vi "akcelerometrWykres.vi"() -> ()   [LabVIEW 2014]
uses:
  <vilib>/MakerHub/LINX/Public/Utilities/Open Local.vi
  <vilib>/MakerHub/LINX/LMH-LINX.lvlib
panel:
  out "deleted portion":dbl[][](array[numeric])
  out "size(s)":i32
  out "Waveform Graph":dbl[][](graph)
  in  "stop":bool
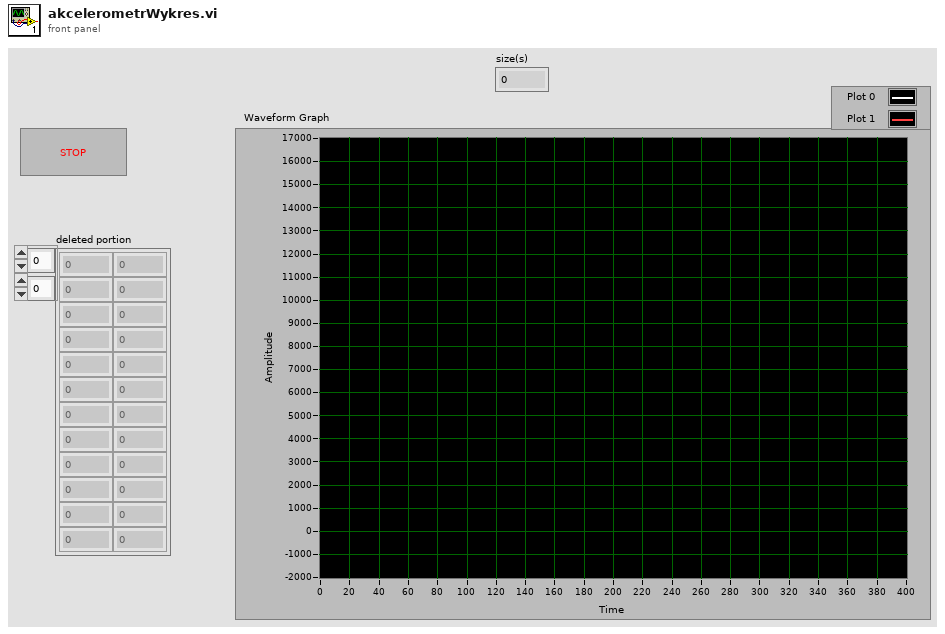
[diagram p1: front panel]
types:
  T1 = typedef "LMH-LINX.lvlib/LINX Ref.ctl" = cluster{"IO":T2, "Interface":T3, "LINX Device Config":T4}
  T2 = typedef "LMH-LINX.lvlib/Platform.ctl" = enum16{"Remote", "Local"}
  T3 = typedef "LMH-LINX.lvlib/Interface.ctl" = enum16{"Serial", "TCP"}
  T4 = typedef "LMH-LINX.lvlib/Device.lvlib/LINX Device Config.ctl" = cluster{"Interface":T3, "COM Port":refnum<visa-resource-name>, "TCP Configuration":T5, "Device Family":u8, "Device ID":u8, "Device Name":string, "TCP Ref":refnum<k5>, "Channels":T6}
  T5 = typedef "LMH-LINX.lvlib/Device.lvlib/TCP Config.ctl" = cluster{"IP Address":string, "Port":u16}
  T6 = typedef "LMH-LINX.lvlib/Channels.ctl" = cluster{"DI":u8[], "DO":u8[], "AI":u8[], "AO":u8[], "PWM":u8[], "QE":u8[], "UART":u8[], "I2C 2":u8[], "SPI":u8[], "CAN":u8[], "Servo":u8[], "AI Ref (V)":dbl, "AI Resolution (Bits)":u8, "AO Ref (V)":dbl, "AO Resolution (Bits)":u8}
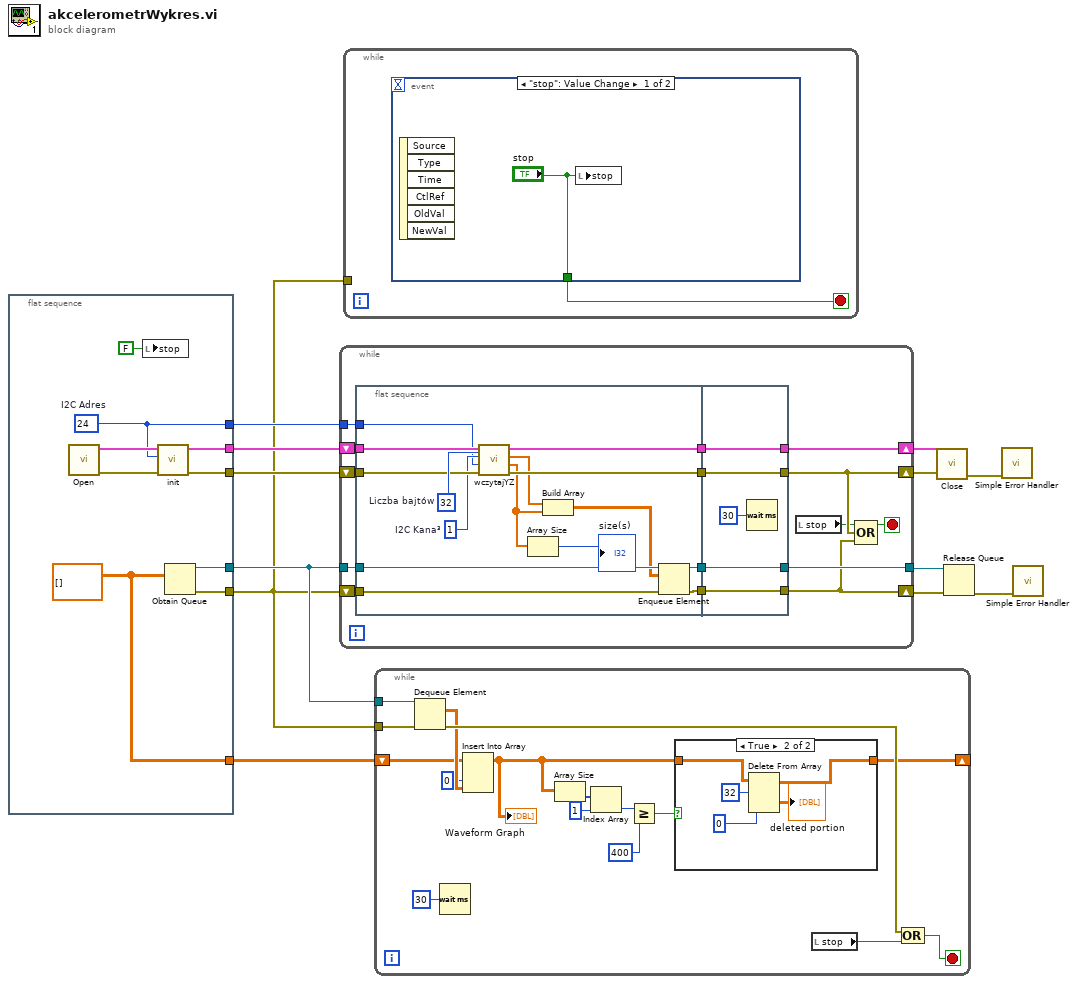
[diagram p0: block diagram]
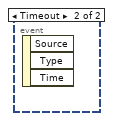
[diagram p2: hidden frame]
diagram:
  n1 = flat-sequence {
    tunnel: [w21] -> w12
    tunnel: [w20] -> w2
    tunnel: [w17] -> w9
    tunnel: [w16] -> w4
    tunnel: [w15] -> w1
    tunnel: [w13] -> w3
    frame #0 {
      w13 = dbl[][] [] ("appended array")
      w17 = u8 24  # I2C Adres
      n2 = call-poly <vilib>:"Open.vi"() -> ("Error Out"=w18:errorcluster, "LINX Resource"=w19:T1)  [unwired: 9 in, 1 out]
      n3 = local write "stop"(FALSE ("stop")) -> ()
      n4 = call "init.vi"("Error In"=w18, "I2C Adres"=w17, "LINX Ref"=w19) -> ("Error Out"=w20:errorcluster, "LINX Resource"=w21:T1)  [unwired: 7 in]
      n5 = Obtain Queue(element data type=w13) -> (queue out=w16:refnum<queue>, error out=w15:errorcluster)  [unwired: 4 in, 1 out]
    }
  }
  n6 = while {
    tunnel: w9 -> [w33]
    shift-right: [w34] -> w11
    shift-left: w12 -> [w36]
    shift-right: [w31] -> w10
    shift-left: w2 -> [w35]
    tunnel: w4 -> [w30]
    tunnel: [w28] -> w7
    shift-right: [w27] -> w6
    shift-left: w1 -> [w29]
    stop <- w32 stop-if-true
    n7 = flat-sequence {
      tunnel: w36 -> [w50]
      tunnel: w35 -> [w49]
      tunnel: w33 -> [w46]
      tunnel: w30 -> [w44]
      tunnel: w29 -> [w43]
      tunnel: [w47] -> w25
      tunnel: [w45] -> w24
      tunnel: [w42] -> w23
      tunnel: [w41] -> w22
      tunnel: [w53] -> w27
      tunnel: [w54] -> w28
      tunnel: [w55] -> w31
      tunnel: [w56] -> w34
      tunnel: w25 -> [w56]
      tunnel: w24 -> [w55]
      tunnel: w23 -> [w54]
      tunnel: w22 -> [w53]
      frame #0 {
        w48 = u8 1  # I2C Kana³
        w51 = u8 32  # Liczba bajtów
        n8 = call "wczytajYZ.vi"("Liczba bajtów"=w51, "error in (no error)"=w49, "I2C Adres"=w46, "I2C Kana³"=w48, "LINX Resource in"=w50) -> ("error out"=w45:errorcluster, "Oœ Z"=w38:dbl[], "Oœ Y"=w39:dbl[], "LINX Resource out"=w47:T1)  [unwired: 3 in]
        n9 = Array Size(array=w38) -> (size(s)=→"size(s)":i32)
        n10 = Build Array(w39, w38) -> (w40:dbl[][])
        n11 = Enqueue Element(queue=w44, element=w40, error in (no error)=w43) -> (queue out=w42:refnum<queue>, error out=w41:errorcluster)  [unwired: 1 in, 1 out]
      }
      frame #1 {
        n12 = Wait (ms)(milliseconds to wait=u32 30 ("millisecond multiple")) -> ()  [unwired: 1 out]
      }
    }
    n13 = local read "stop"() -> (w26:bool)
    n14 = Compound Arithmetic op=OR(w26, w31, w27) -> (w32:bool)
  }
  n15 = while {
    tunnel: w1 -> [_]
    stop <- w57 stop-if-true
    n16 = event shown="[0] \"stop\": Value Change" {
      selector: _ -> [_ _]
      dyn-events: _ -> [_ _]
      timeout: _ -> [_ _]
      tunnel: ["stop" _] -> w57
      event "stop": Value Change {
        n17 = event-data() -> ()  [unwired: 1 in, 6 out]
        n18 = local write "stop"("stop") -> ()
      }
      event Timeout {
        n19 = event-data() -> ()  [unwired: 1 in, 3 out]
      }
    }
  }
  n20 = while {
    tunnel: w4 -> [w74]
    tunnel: w1 -> [w73]
    shift-right: [w66] -> _
    shift-left: w3 -> [w68]
    stop <- w71 stop-if-true
    n21 = Dequeue Element(queue=w74, error in (no error)=w73) -> (element=w69:dbl[][], error out=w70:errorcluster)  [unwired: 1 in, 2 out]
    n22 = Wait (ms)(milliseconds to wait=u32 30 ("millisecond multiple")) -> ()  [unwired: 1 out]
    n23 = Insert Into Array(array=w68, index (col)=0 ("disabled index (col)"), new element=w69) -> (w67:dbl[][])  [unwired: 1 in]
    "Waveform Graph" <- w67
    n24 = Array Size(array=w67) -> (size(s)=w65:i32[])
    n25 = Index Array(array=w65, index=1) -> (element=w64:i32)
    n26 = Greater Or Equal?(x=w64, y=400) -> (x >= y?=w62:bool)
    n27 = case shown="True" w62 {
      tunnel: w67 -> [w75 w80]
      tunnel: [w75 w79] -> w66
      frame False {
      }
      frame True {
        n28 = Delete From Array(array=w80, length=32, index (row)=0) -> (deleted portion=→"deleted portion":dbl[][], array with subset deleted=w79:dbl[][])  [unwired: 1 in]
      }
    }
    n29 = local read "stop"() -> (w72:bool)
    n30 = Compound Arithmetic op=OR(w70, w72) -> (w71:bool)
  }
  n31 = call <vilib>:"Close.vi"("Error In"=w10, "LINX Resource"=w11) -> ("Error Out"=w8:errorcluster)  [unwired: 9 in]
  n32 = Release Queue(queue=w7, error in (no error)=w6) -> (error out=w5:errorcluster)  [unwired: 1 in, 2 out]
  n33 = call <vilib>:"Simple Error Handler.vi"("error in (no error)"=w8) -> ()  [unwired: 4 in, 5 out]
  n34 = call <vilib>:"Simple Error Handler.vi"("error in (no error)"=w5) -> ()  [unwired: 4 in, 5 out]
